vi "DriveStraightCalculations.vi"(8 "error in (no error)":errorcluster, 11 "DriveBase.lvclass":refnum<class "DriveBase.lvclass">) -> (0 "error out":errorcluster, 2 "PIDOutput":dbl, 3 "DriveBase.lvclass":refnum<class "DriveBase.lvclass">)   [LabVIEW 2016, in "DriveBase.lvclass"]
uses:
  DriveBase.lvclass
  <vilib>/addons/control/pid/pid.llb/PID (DBL).vi
  <vilib>/addons/control/pid/NI_PID_pid.lvlib
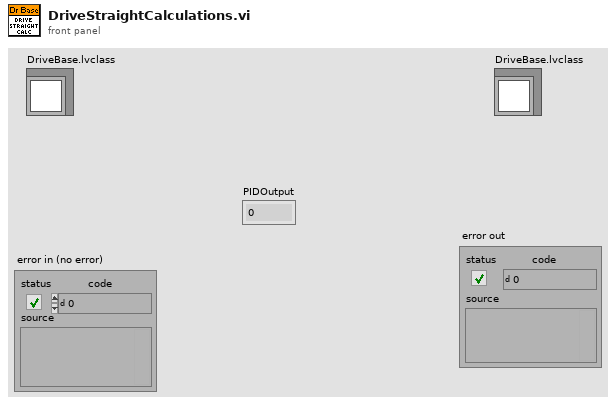
[diagram p1: front panel]
types:
  T1 = cluster{"proportional gain (Kc)":dbl, "integral time (Ti, min)":dbl, "derivative time (Td, min)":dbl}
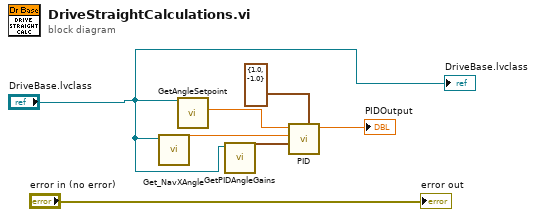
[diagram p0: block diagram]
diagram:
  n1 = call-dynamic "Get_NavXAngle.vi"("DriveBase in"="DriveBase.lvclass") -> ("NavX Angle"=w7:dbl)  [unwired: 9 in, 1 out]
  n2 = call "GetAngleSetpoint.vi"("DriveBase.lvclass"="DriveBase.lvclass") -> ("angleSepointOutput"=w4:dbl)  [unwired: 9 in, 1 out]
  n3 = call "GetPIDAngleGains.vi"("DriveBase.lvclass"="DriveBase.lvclass") -> ("Angle PID gains"=w6:T1)  [unwired: 9 in, 1 out]
  n4 = call-poly <vilib>:"PID.vi"("output range"=cluster{"output high":dbl, "output low":dbl} {"output high"=1.0, "output low"=-1.0}, "PID gains"=w6, "process variable"=w7, "setpoint"=w4) -> ("output"=→"PIDOutput":dbl)  [unwired: 6 in, 1 out]
  "DriveBase.lvclass" <- "DriveBase.lvclass"
  "error out" <- "error in (no error)"
